vi "Resistivity Calculate Q.vi"(8 "error in (no error)":errorcluster, 11 "V1-V8 VDP":dbl[](array[numeric])) -> (0 "error out":errorcluster, 1 "QB":dbl, 3 "QA":dbl)   [LabVIEW 2016, in "Hall Effect Library.lvlib"]
uses:
  Hall Effect Library.lvlib
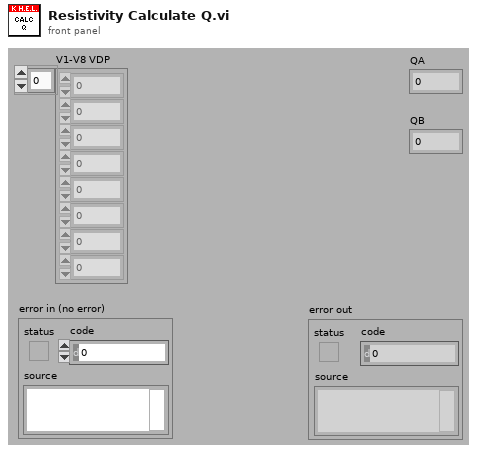
[diagram p1: front panel]
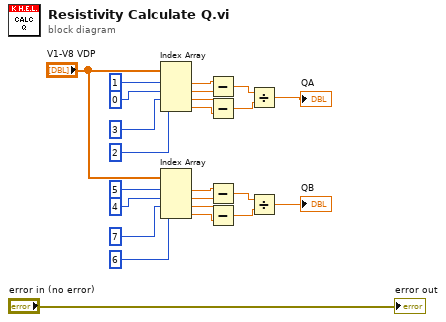
[diagram p0: block diagram]
diagram:
  n1 = Index Array(array="V1-V8 VDP", index #1=1 ("index"), index #2=0 ("index"), index #3=3 ("index"), index #4=2 ("index")) -> (element #1=w20:dbl, element #2=w19:dbl, element #3=w18:dbl, element #4=w17:dbl)
  n2 = Index Array(array="V1-V8 VDP", index #1=5 ("index"), index #2=4 ("index"), index #3=7 ("index"), index #4=6 ("index")) -> (element #1=w7:dbl, element #2=w8:dbl, element #3=w9:dbl, element #4=w10:dbl)
  n3 = Subtract(x=w20, y=w19) -> (x-y=w16:dbl)
  n4 = Subtract(x=w18, y=w17) -> (x-y=w15:dbl)
  n5 = Subtract(x=w7, y=w8) -> (x-y=w11:dbl)
  n6 = Subtract(x=w9, y=w10) -> (x-y=w12:dbl)
  n7 = Divide(x=w16, y=w15) -> (x/y=→"QA":dbl)
  n8 = Divide(x=w11, y=w12) -> (x/y=→"QB":dbl)
  "error out" <- "error in (no error)"
